vi "get_control_image.vi"() -> ()   [LabVIEW 2021]
panel:
  out "2D Picture":picture
  in  "Multicolumn Listbox":i32(listbox)
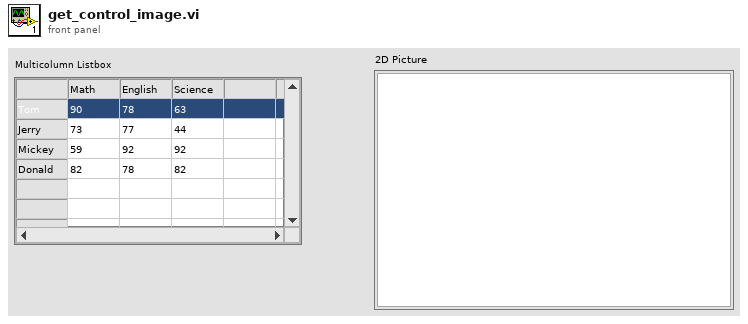
[diagram p1: front panel]
types:
  T1 = typedef "imagedata.ctl" = cluster{"image type":i32, "image depth":i32, "image":u8[], "mask":u8[], "colors":u32[], "Rectangle":cluster{"left":i16, "top":i16, "right":i16, "bottom":i16}}
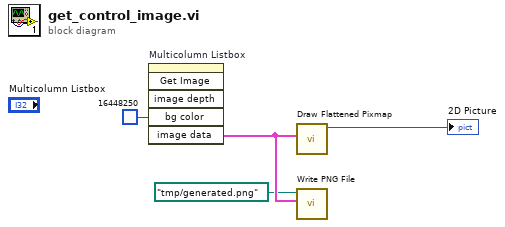
[diagram p0: block diagram]
diagram:
  n1 = invoke on="Multicolumn Listbox" class="MCListbox (strict)" method="Get Image"("bg color"=u32 16448250 ("Background Color")) -> ("image data"=w2:T1)  [unwired: 5 in, 5 out]
  n2 = call <vilib>:"Draw Flattened Pixmap.vi"("image data"=w2) -> ("new picture"=→"2D Picture":picture)  [unwired: 8 in]
  n3 = call <vilib>:"Write PNG File.vi"("image data"=w2, "path to PNG file"=path "/tmp/generated.png") -> ()  [unwired: 8 in, 2 out]
